vi "Integer Vector.vi"() -> (0 "error out":errorcluster, 3 "Passed?":bool)   [LabVIEW 2009]
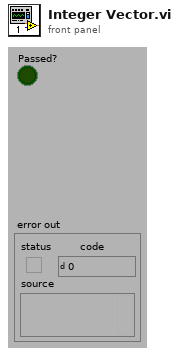
[diagram p1: front panel]
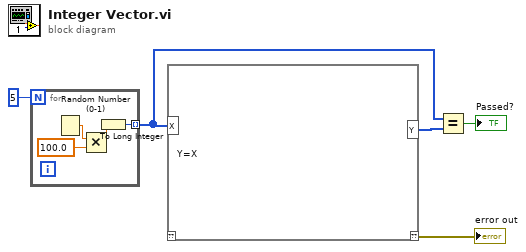
[diagram p0: block diagram]
diagram:
  n1 = for {
    N: 5 -> [_]
    tunnel: [w8] -> w2 mode=indexing
    n2 = Random Number (0-1)() -> (number: 0 to 1=w9:dbl)
    n3 = Multiply(x=w9, y=100.0) -> (x*y=w7:dbl)
    n4 = To Long Integer(number=w7) -> (32bit integer=w8:i32)
  }
  n5 = script code="Y=X"("X"=w2) -> ("??"=→"error out":errorcluster, "Y"=w1:i32[])  [unwired: 1 in]
  n6 = Equal?(x=w2, y=w1) -> (x = y?=→"Passed?":bool)
